vi "Test_PublicationLocked_PublisherNotOwner_Reject.vi"(8 "error in (no error)":errorcluster, 11 "TestMediator In":refnum<class "TestMediationSemantics.lvclass">) -> (0 "error out":errorcluster, 3 "TestMediator Out":refnum<class "TestMediationSemantics.lvclass">)   [LabVIEW 2017, in "TestMediationSemantics.lvclass"]
uses:
  TestMediationSemantics.lvclass
  Source/Framework/Mediator/Mediator/Mediator.lvclass
  C:/Program Files (x86)/National Instruments/LabVIEW 2017/vi.lib/ActorFramework/Actor/Actor.lvclass
  Source/Framework/IMediator/PublishRequest/PublishRequest.lvclass/PublishRequest.ctl
  Source/Framework/SubscriptionPolicy/BasicSubscription/BasicSubscription.lvclass/BasicSubscription.ctl
  Source/Framework/IMediator/SubscriptionRequest/SubscriptionRequest.lvclass/SubscriptionRequest.ctl
  Source/Framework/IMediator/IMediator Messages/Lock Publication Msg/Lock Publication Msg.lvclass/Lock Publication Msg.ctl
  <vilib>/ActorFramework/Message Enqueuer/Message Enqueuer.lvclass/Message Enqueuer.ctl
  Source/Framework/IMediator/IMediator Messages/Publish Msg/Publish Msg.lvclass/Publish Msg.ctl
  Source/Framework/IMediator/IMediator Messages/Subscribe Msg/Subscribe Msg.lvclass/Subscribe Msg.ctl
  gpm_packages/@cs/transport/Source/Concrete/QueueTransport/QueueTransport.lvclass/QueueTransport.ctl
  <vilib>/ActorFramework/Message Enqueuer/Enqueue.vi
  Source/Framework/SubscriptionPolicy/BasicSubscription/BasicSubscription.lvclass
  C:/Git/mva-framework/Source/Framework/IMediator/ISubscriptionPolicy/ISubscriptionPolicy.lvclass
  Source/Framework/IMediator/IMediator Messages/Lock Publication Msg/Lock Publication Msg.lvclass
  C:/Program Files (x86)/National Instruments/LabVIEW 2017/vi.lib/ActorFramework/Message/Message.lvclass
  Source/Framework/IMediator/IMediator Messages/Publish Msg/Publish Msg.lvclass
  gpm_packages/@cs/transport/Source/Concrete/QueueTransport/QueueTransport.lvclass
  C:/Git/mva-framework/gpm_packages/@cs/transport/Source/ITransport/ITransport.lvclass
  Source/Framework/IMediator/IMediator Messages/Subscribe Msg/Subscribe Msg.lvclass
  <vilib>/ActorFramework/Stop Msg/Stop Msg.lvclass
  <vilib>/Utility/error.llb/Error Cluster From Error Code.vi
  <vilib>/ActorFramework/Message Priority Queue/Priority Enqueue.vi
  Source/Framework/IMediator/SubscriptionRequest/SubscriptionRequest.lvclass
  Source/Framework/IMediator/IPublicationPolicy/IPublicationPolicy.lvclass
  gpm_packages/@cs/transport/Source/ITransport/ITransport.lvclass
  Source/Framework/IMediator/PublishRequest/PublishRequest.lvclass
  <vilib>/ActorFramework/Actor/Actor.lvclass
  Source/Framework/IMediator/ISubscriptionPolicy/ISubscriptionPolicy.lvclass
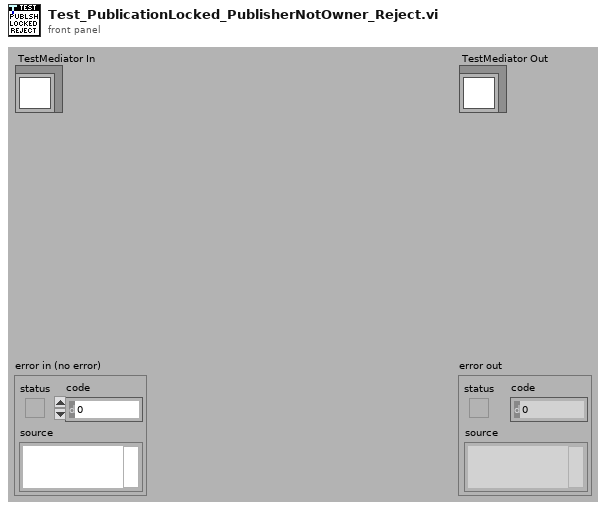
[diagram p1: front panel]
types:
  T1 = typedef "IMediator.lvlib/ISubscriptionPolicy.lvclass/ISubscriptionPolicy Reference.ctl" = refnum<data-value>
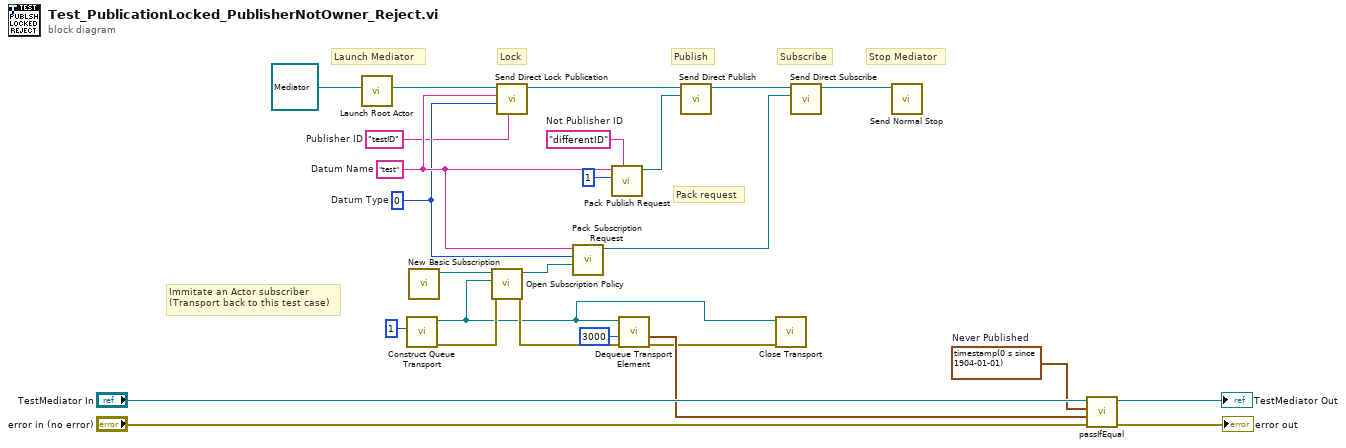
[diagram p0: block diagram]
diagram:
  w3 = timestamp(0 s since 1904-01-01)  # Never Published
  w5 = "differentID"  # Not Publisher ID
  w6 = "testID"  # Publisher ID
  w7 = 0  # Datum Type
  w8 = "test"  # Datum Name
  # "Immitate an Actor subscriber\n(Transport back to this test case)"
  # "Pack request"
  # "Lock"
  # "Launch Mediator"
  # "Stop Mediator"
  # "Subscribe"
  # "Publish"
  n1 = call <vilib>:"Launch Root Actor.vi"("Actor"=refnum<class "Mediator.lvclass"> refnum ("Mediator.lvlib:Mediator.lvclass")) -> ("Actor's Enqueuer"=w21:refnum<class "Message Enqueuer.lvclass">)  [unwired: 9 in, 1 out]
  n2 = call "Construct Queue Transport.vi"("Max Queue Size (-1)"=1) -> ("error out"=w16:errorcluster, "QueueTransport"=w2:refnum<class "QueueTransport.lvclass">)  [unwired: 9 in]
  n3 = call "New Basic Subscription.vi"() -> ("BasicSubscription Out"=w13:refnum<class "BasicSubscription.lvclass">)  [unwired: 11 in]
  n4 = call "Open Subscription Policy.vi"("error in (no error)"=w16, "Transport"=w2, "SubscriptionPolicy"=w13) -> ("error out"=w15:errorcluster, "Subscription Policy"=w12:T1)  [unwired: 7 in]
  n5 = call "Send Direct Lock Publication.vi"("Publisher ID"=w6, "Datum Type"=w7, "Datum Name"=w8, "Mediator Enqeuer"=w21) -> ("Mediator Enqueuer out"=w9:refnum<class "Message Enqueuer.lvclass">)  [unwired: 6 in, 1 out]
  n6 = call "Pack Subscription Request.vi"("Subscription Policy"=w12, "Type"=w7, "Datum Name"=w8) -> ("SubscriptionRequest"=w20:refnum<class "SubscriptionRequest.lvclass">)  [unwired: 8 in]
  n7 = call "Pack Publish Request.vi"("Publisher ID"=w5, "Data to Publish"=1, "Datum Name"=w8) -> ("PublishRequest"=w10:refnum<class "PublishRequest.lvclass">)  [unwired: 8 in]
  n8 = call "Dequeue Transport Element.vi"("error in (no error)"=w15, "Timeout In ms (-1)"=3000, "QueueTransport"=w2) -> ("error out"=w1:errorcluster, "Publication Time"=w4:timestamp)  [unwired: 5 in, 2 out]
  n9 = call "Send Direct Publish.vi"("PublishRequest"=w10, "Mediator Enqeuer"=w9) -> ("Mediator Enqueuer out"=w19:refnum<class "Message Enqueuer.lvclass">)  [unwired: 8 in, 1 out]
  n10 = call-dynamic "Close Transport.vi"("error in (no error)"=w1, "QueueTransport"=w2) -> ()  [unwired: 9 in, 1 out]
  n11 = call "Send Direct Subscribe.vi"("Subscription Request"=w20, "Message Enqueuer"=w19) -> ("Message Enqueuer out"=w14:refnum<class "Message Enqueuer.lvclass">)  [unwired: 8 in, 1 out]
  n12 = call <vilib>:"Send Normal Stop.vi"("Message Enqueuer"=w14) -> ()  [unwired: 10 in, 1 out]
  n13 = call-dynamic "passIfEqual.vi"("error in (no error)"="error in (no error)", "y"=w4, "x"=w3, "TestCase in"="TestMediator In") -> ("error out"=→"error out":errorcluster, "TestCase out"=→"TestMediator Out":refnum<class "TestMediationSemantics.lvclass">)  [unwired: 6 in]
